vi "BSCAN_DEMO06_IMX8_I2C_PCA9450.vi"() -> ()   [LabVIEW 2017]
uses:
  Saldigi_protocol_library.lvlibp/I2C_bitstream/I2C_typedef.ctl
  Saldigi_protocol_library.lvlibp/HAL/HAL_version_typedef.ctl
  Saldigi_protocol_library.lvlibp/Drivers/PCA9450_typedef.ctl
  Saldigi_protocol_library.lvlibp
panel:
  in  "stop":bool
  out "error out":errorcluster
  in  "I2C typedef in":T1={"SDA padded"=[], "CLK padded"=[], "String array"=[], "Slave addr 7bit"=37, "clocked bits"=0, "output rate"=0.0, "SDA channel name"="chain0/IMX8MMINI-BSDL/I2C1_SDA", "CLK channel name"="chain0/IMX8MMINI-BSDL/I2C1_SCL", "SDA-IN channel name"="", "Version"=enum."BSCAN V2", "Parameter string"="PFI5"} {"Slave addr 7bit" format="%07b"}
  out "PCA9450 Register value out":u8 format="%.0x"
  out "dt":dbl=0.015491600000132166
  # "saldigi.fi protocol library"
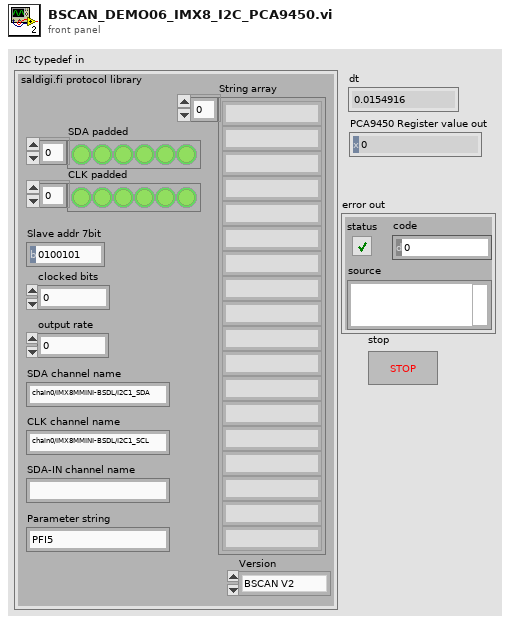
[diagram p1: front panel]
types:
  T1 = typedef "Saldigi_protocol_library.lvlibp/I2C_typedef.ctl" = cluster{"SDA padded":bool[], "CLK padded":bool[], "String array":string[], "Slave addr 7bit":u8, "clocked bits":i32, "output rate":dbl, "SDA channel name":string, "CLK channel name":string, "SDA-IN channel name":string, "Version":T2, "Parameter string":string}
  T2 = typedef "Saldigi_protocol_library.lvlibp/HAL_version_typedef.ctl" = enum16{"DAQmx V1", "DAQmx V2", "FTn232H", "BSCAN V1", "DAQmx V1.1", "DAQmx V2.1", "J-LINK BSCAN", "BSCAN V2"}
  T3 = typedef "Saldigi_protocol_library.lvlibp/PCA9450_typedef.ctl" = enum16{"Device_ID"}
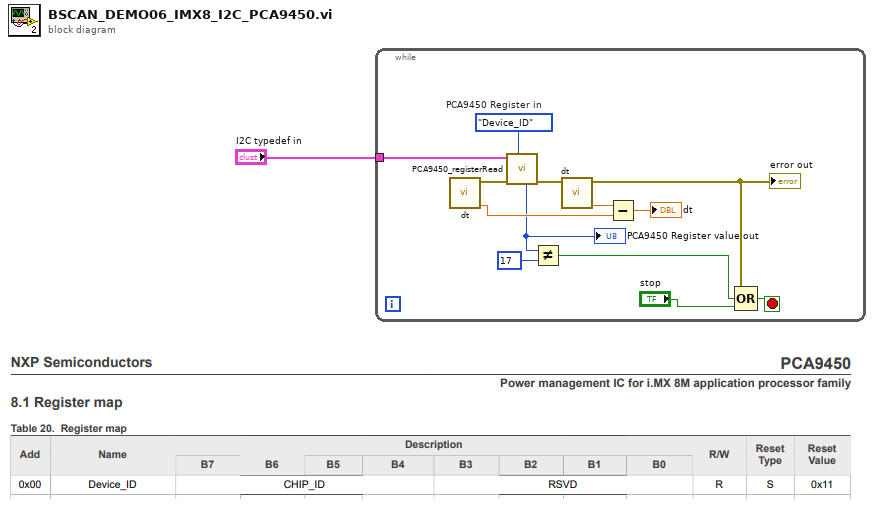
[diagram p0: block diagram]
diagram:
  n1 = while {
    tunnel: "I2C typedef in" -> [w12]
    stop <- w8 stop-if-true
    w13 = PCA9450_typedef."Device_ID"  # PCA9450 Register in
    n2 = call "dt.vi"() -> ("relative seconds"=w10:dbl, "error out"=w11:errorcluster)  [unwired: 10 in]
    n3 = call "PCA9450_registerRead.vi"("PCA9450 Register in"=w13, "error in"=w11, "I2C typedef in"=w12) -> ("error out"=w4:errorcluster, "PCA9450 Register value out"=w7:u8)  [unwired: 6 in, 1 out]
    "PCA9450 Register value out" <- w7
    n4 = Not Equal?(x=w7, y=u8 17) -> (x != y?=w5:bool)
    n5 = call "dt.vi"("error in"=w4) -> ("relative seconds"=w9:dbl, "error out"=w2:errorcluster)  [unwired: 9 in]
    "error out" <- w2
    n6 = Subtract(x=w9, y=w10) -> (x-y=→"dt":dbl)
    n7 = Compound Arithmetic op=OR(w2, w5, "stop") -> (w8:bool)
  }
